vi "表格快捷菜单输入单元格.vi"() -> ()   [LabVIEW 2013, in "Table Tool.lvlib"]
uses:
  Table Tool.lvlib
  <vilib>/Utility/miscctls.llb/LVRowAndColumnTypeDef.ctl
panel:
  in  "停止按钮":bool
  out "选择人物":string[][](table)
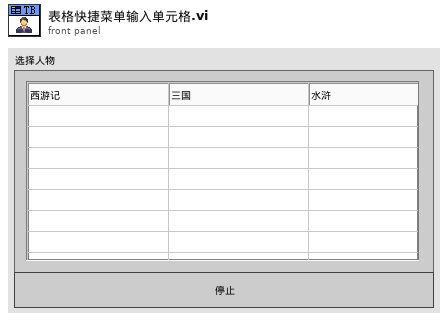
[diagram p1: front panel]
types:
  T1 = typedef "LVRowAndColumnTypeDef.ctl" = cluster{"Row":i32, "Column":i32}
  T2 = typedef "LVPoint32TypeDef.ctl" = cluster{"Horizontal":i32, "Vertical":i32}
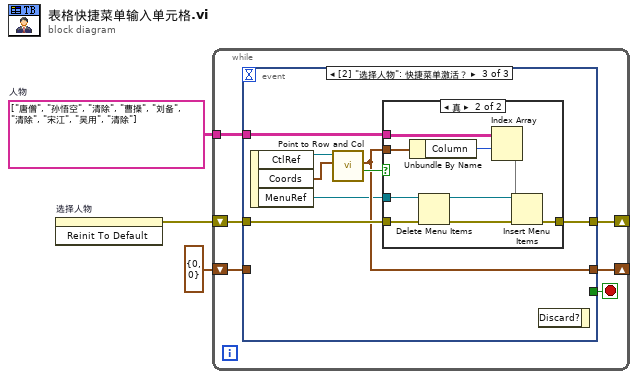
[diagram p0: block diagram]
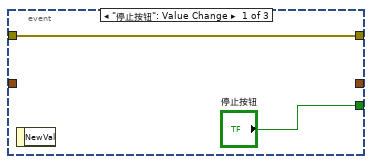
[diagram p2: hidden frame]
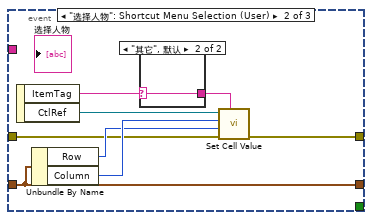
[diagram p3: hidden frame]
diagram:
  w2 = string[][] [["唐僧", "孙悟空", "清除"], ["曹操", "刘备", "清除"], ["宋江", "吴用", "清除"]]  # 人物
  n1 = invoke on="选择人物" class="Tbl (严格)" method="Reinit To Default"() -> (error out=w3:errorcluster)  [unwired: 3 in, 2 out]
  n2 = while {
    shift-right: [w6] -> _
    shift-left: w3 -> [w8]
    tunnel: w2 -> [w7]
    shift-right: [w5] -> _
    shift-left: T1 {"Row"=0, "Column"=0} ("单元格位置") -> [w4]
    stop <- w9 stop-if-true
    n3 = event shown="[2] \"选择人物\": 快捷菜单激活？" {
      selector: _ -> [_ _ _]
      dyn-events: _ -> [_ _ _]
      timeout: _ -> [_ _ _]
      tunnel: ["停止按钮" _ _] -> w9
      tunnel: w8 -> [w10 w12 w25]
      tunnel: w7 -> [_ _ w23]
      tunnel: [w10 w13 w24] -> w6
      tunnel: [_ w19 w22] -> w5
      tunnel: w4 -> [_ w19 _]
      event "停止按钮": Value Change {
        n4 = event-data() -> ()  [unwired: 1 in, 1 out]
      }
      event "选择人物": Shortcut Menu Selection (User) {
        n5 = event-data() -> ("ItemTag"=w18:string, "CtlRef"=w16:refnum<vi>)  [unwired: 1 in]
        n6 = Unbundle By Name(w19) -> ("Row"=w14:i32, "Column"=w15:i32)
        n7 = case shown="\"其它\", 默认" w18 {
          selector: w18 -> [_ w20]
          tunnel: [_ w20] -> w17
          frame "清除" {
          }
          frame "其它", Default {
          }
        }
        n8 = call "Set Cell Value.vi"("值"=w17, "error in (no error)"=w12, "Y索引"=w14, "X索引"=w15, "Table Ref In"=w16) -> ("error out"=w13:errorcluster)  [unwired: 5 in, 1 out]
      }
      event "选择人物": Shortcut Menu Activation? {
        n9 = event-data() -> ("CtlRef"=w28:refnum<vi>, "Coords"=w27:T2, "MenuRef"=w21:refnum<k9>)  [unwired: 1 in]
        n10 = call "Point to Row and Col.vi"("点"=w27, "Table Ref In"=w28) -> ("边界内？"=w26:bool, "单元格位置"=w22:T1)  [unwired: 6 in, 2 out]
        n11 = case shown="真" w26 {
          tunnel: w22 -> [_ w32]
          tunnel: w25 -> [w29 w38]
          tunnel: [w29 w31] -> w24
          tunnel: w23 -> [_ w35]
          tunnel: w21 -> [_ w30]
          frame False {
          }
          frame True {
            n12 = Unbundle By Name(w32) -> ("Column"=w36:i32)
            n13 = Delete Menu Items(6:w38, 9:w30) -> (0:w37:errorcluster, 3:w33:refnum<k9>)  [unwired: 2 out]
            n14 = Index Array(array=w35, index (row)=w36) -> (element=w34:string[])  [unwired: 1 in]
            n15 = Insert Menu Items(6:w37, 8:w34, 9:w33) -> (0:w31:errorcluster)  [unwired: 5 out]
          }
        }
        n16 = event-data() -> ()  [unwired: 2 in, 1 out]
      }
    }
  }
